vi "Timer Control Example.vi"() -> ()   [LabVIEW 2011]
panel:
  out "Total time (s)":dbl format="%.3f"
  in  "Exit":bool
  out "Running":bool
  in  "Reset Timer":bool
  in  "Stop Timer":bool
  in  "Start Timer":bool
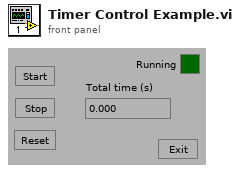
[diagram p1: front panel]
types:
  T1 = typedef "Timer Refnum.ctl" = refnum<k1>
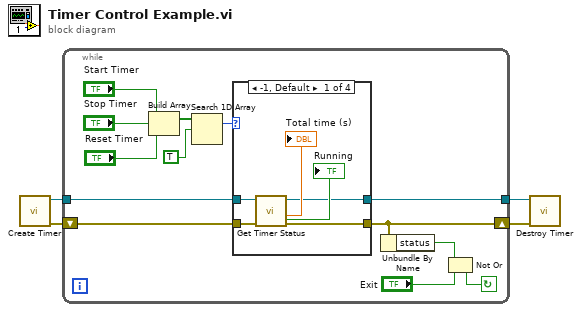
[diagram p0: block diagram]
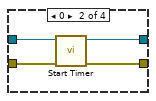
[diagram p2: hidden frame]
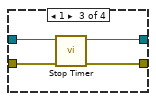
[diagram p3: hidden frame]
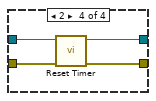
[diagram p4: hidden frame]
diagram:
  n1 = call "Create Timer.vi"() -> ("error out"=w3:errorcluster, "timer"=w4:T1)  [unwired: 5 in, 1 out]
  n2 = while {
    tunnel: [w5] -> w2
    shift-left: w3 -> [w10]
    shift-right: [w9] -> w1
    tunnel: w4 -> [w11]
    stop <- w6 continue-if-true
    n3 = Build Array("Start Timer", "Stop Timer", "Reset Timer") -> (w14:bool[])
    n4 = Search 1D Array(1D array=w14, element=TRUE) -> (index of element=w12:i32)  [unwired: 1 in]
    n5 = case shown="-1, Default" w12 {
      tunnel: w11 -> [w21 w27 w31 w35]
      tunnel: w10 -> [w20 w26 w30 w34]
      tunnel: [w19 w24 w28 w32] -> w9
      tunnel: [w18 w25 w29 w33] -> w5
      frame -1, Default {
        n6 = call "Get Timer Status.vi"("error in (no error)"=w20, "timer"=w21) -> ("error out"=w19:errorcluster, "Total time (s)"=→"Total time (s)":dbl, "timer out"=w18:T1, "Running"=→"Running":bool)  [unwired: 4 in, 2 out]
      }
      frame 0 {
        n7 = call "Start Timer.vi"("error in (no error)"=w26, "timer"=w27) -> ("error out"=w24:errorcluster, "timer out"=w25:T1)  [unwired: 8 in]
      }
      frame 1 {
        n8 = call "Stop Timer.vi"("error in (no error)"=w30, "timer"=w31) -> ("error out"=w28:errorcluster, "timer out"=w29:T1)  [unwired: 8 in]
      }
      frame 2 {
        n9 = call "Reset Timer.vi"("error in (no error)"=w34, "timer"=w35) -> ("error out"=w32:errorcluster, "timer out"=w33:T1)  [unwired: 8 in]
      }
    }
    n10 = Unbundle By Name(w9) -> ("status"=w8:bool)
    n11 = Not Or(1:"Exit", 2:w8) -> (0:w6:bool)
  }
  n12 = call "Destroy Timer.vi"("error in (no error)"=w1, "timer"=w2) -> ()  [unwired: 4 in, 2 out]
